vi "Get DAQmx DI Task Ref from DI TaskName.vi"(8 "error in (no error)":errorcluster, 10 "AI TaskName":string, 11 "DAQ":refnum<class "DAQ.lvclass">) -> (0 "error out":errorcluster, 2 "DAQmx DI Task":refnum<k21>, 3 "DAQ":refnum<class "DAQ.lvclass">)   [LabVIEW 2017, in "DAQ.lvclass"]
doc: "Developed by Kevin Thompson\nkevin@thompsonengineering.net\n\nCopyright 2018-2020\nThompson Engineering, LLC"
uses:
  DAQ.lvclass
  DAQ.lvclass/DAQ.ctl
  DataTypes/TD DI TaskIO.ctl
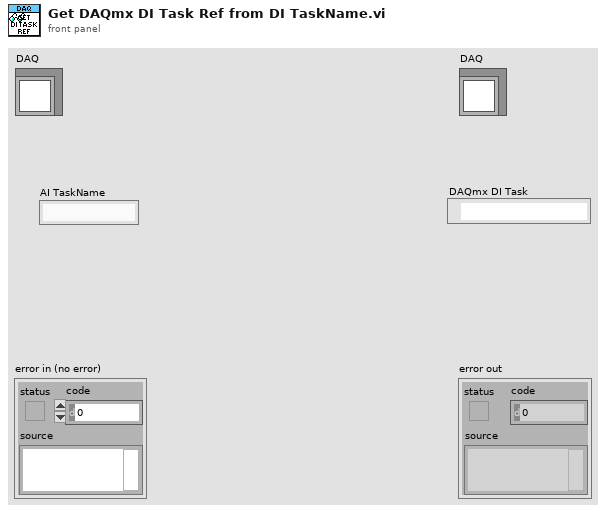
[diagram p1: front panel]
types:
  T1 = typedef "DAQ.lvclass/TD DI TaskIO.ctl" = cluster{"DI TaskName":string, "IONames":string[], "DAQmxDI TaskRef":refnum<k21>}
  T2 = typedef "TD Dynamic CVT DVR--ref.ctl" = refnum<data-value>
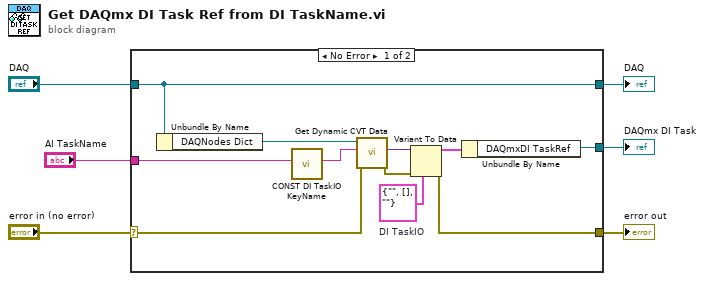
[diagram p0: block diagram]
diagram:
  n1 = case shown="No Error" "error in (no error)" {
    selector: "error in (no error)" -> [w15 w18]
    tunnel: [w14 w18] -> w5
    tunnel: [w17 w19] -> w3
    tunnel: "DAQ" -> [w17 w19]
    tunnel: "AI TaskName" -> [w9 _]
    tunnel: [w10 _] -> w1
    frame No Error {
      w7 = T1 {"DI TaskName"="", "IONames"=[], "DAQmxDI TaskRef"=""}  # DI TaskIO
      n2 = Unbundle By Name(w17) -> ("DAQNodes Dict"=w16:T2)
      n3 = call "CONST DI TaskIO KeyName.vi"("DI TaskName"=w9) -> ("DI TaskIO (KeyName)"=w8:string)  [unwired: 10 in]
      n4 = call <vilib>:"Get Dynamic CVT Data.vi"("error in (no error)"=w15, "DataName"=w8, "dCVT DVR"=w16) -> ("error out"=w13:errorcluster, "value"=w12:variant)  [unwired: 5 in, 2 out]
      n5 = Variant To Data(error in=w13, type=w7, Variant=w12) -> (data=w11:T1, error out=w14:errorcluster)
      n6 = Unbundle By Name(w11) -> ("DAQmxDI TaskRef"=w10:refnum<k21>)
    }
    frame Error {
    }
  }
  "error out" <- w5
  "DAQ" <- w3
  "DAQmx DI Task" <- w1
